vi "acelerometro.vi"(0 "Handle table":string[][](array[string]), 5 "COM Bluegiga in":refnum<visa-resource-name>, 7 "Service UUID":string, 9 "error in (no error)":errorcluster, 11 "Characteristic UUID":string, 12 "Connection Status":T1={"MAC Address"="", "cnx handle"=0, "cnx flags"=0, "Address Type"=125, "Connection Interval (ms)"=125, "Timeout(ms)"=125, "Latency"=0, "bonding handle"=0} {"Address Type" items=["Public", "Random"]}) -> (1 "error out":errorcluster, 3 "COM Bluegiga out":refnum<visa-resource-name>, 6 "z (acel)":dbl, 10 "y (acel)":dbl, 15 "x (acel)":dbl)   [LabVIEW 2020]
uses:
  <vilib>/BLE/type_def/connection_status_bundle.ctl
  <vilib>/BLE/type_def/address_type.ctl
panel:
  out "characteristic value":u8[](array[numeric])
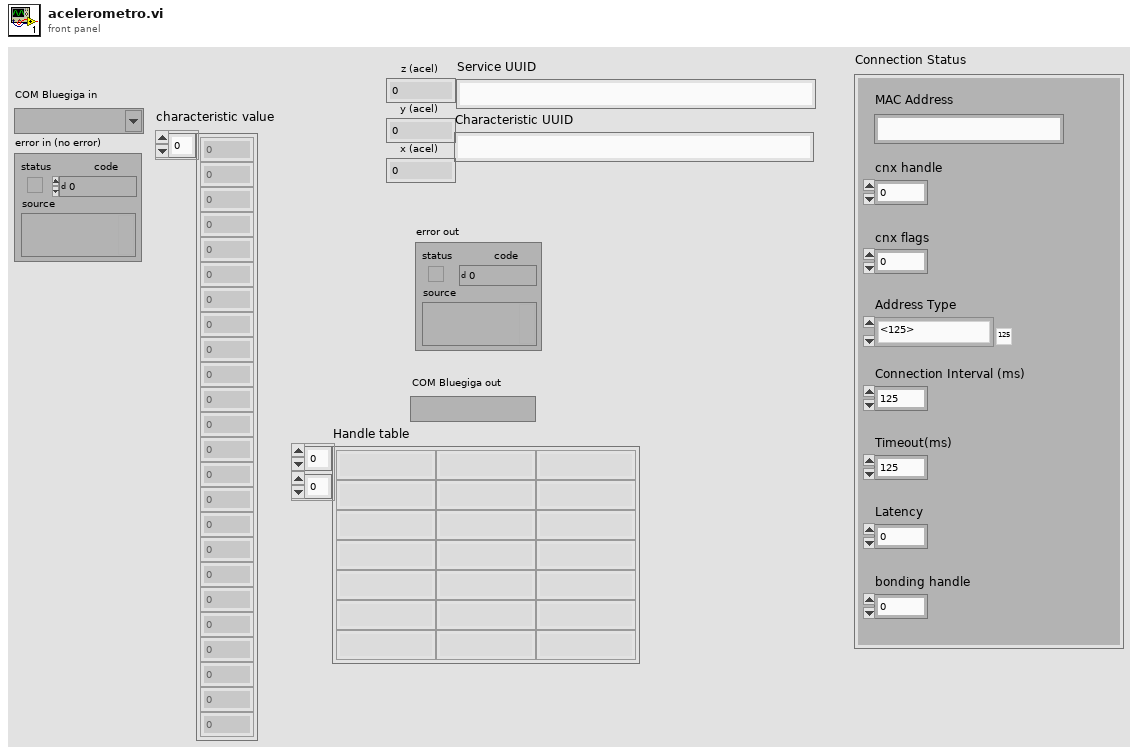
[diagram p1: front panel]
types:
  T1 = typedef "connection_status_bundle.ctl" = cluster{"MAC Address":string, "cnx handle":u8, "cnx flags":u8, "Address Type":T2, "Connection Interval (ms)":u16, "Timeout(ms)":u16, "Latency":u16, "bonding handle":u8}
  T2 = typedef "address_type.ctl" = u8
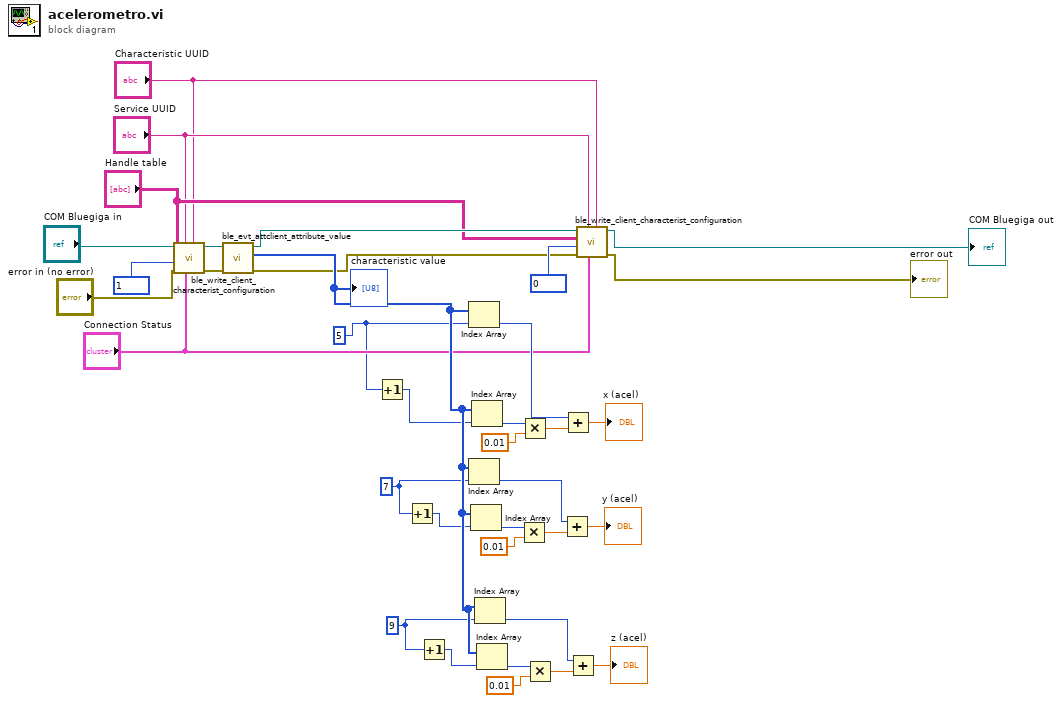
[diagram p0: block diagram]
diagram:
  w1 = 9 ("y")
  w2 = 7 ("y")
  w5 = 5 ("y")
  n1 = call <vilib>:"ble_write_client_characterist_configuration.vi"("Characteristic UUID"="Characteristic UUID", "Connection Status"="Connection Status", "Service UUID"="Service UUID", "error in (no error)"="error in (no error)", "Value(16bit)"=u16 1, "Handle table"="Handle table", "COM Bluegiga in"="COM Bluegiga in") -> ("error out"=w18:errorcluster, "COM Bluegiga out"=w17:refnum<visa-resource-name>)  [unwired: 3 in]
  n2 = call <vilib>:"ble_evt_attclient_attribute_value.vi"("error in (no error)"=w18, "COM Bluegiga in"=w17) -> ("error out"=w13:errorcluster, "characteristic value"=w21:u8[], "COM Bluegiga out"=w14:refnum<visa-resource-name>)  [unwired: 6 in, 1 out]
  "characteristic value" <- w21
  n3 = Increment(x=w5) -> (x+1=w6:i32)
  n4 = Increment(x=w2) -> (x+1=w3:i32)
  n5 = Increment(x=w1) -> (x+1=w4:i32)
  n6 = Index Array(array=w21, index=w5) -> (element=w33:u8)
  n7 = Index Array(array=w21, index=w2) -> (element=w27:u8)
  n8 = Index Array(array=w21, index=w3) -> (element=w28:u8)
  n9 = Index Array(array=w21, index=w6) -> (element=w36:u8)
  n10 = Index Array(array=w21, index=w1) -> (element=w22:u8)
  n11 = Index Array(array=w21, index=w4) -> (element=w23:u8)
  n12 = Multiply(x=w28, y=0.01) -> (x*y=w30:dbl)
  n13 = Multiply(x=w36, y=0.01) -> (x*y=w34:dbl)
  n14 = Multiply(x=w23, y=0.01) -> (x*y=w25:dbl)
  n15 = Add(x=w27, y=w30) -> (x+y=→"y (acel)":dbl)
  n16 = Add(x=w33, y=w34) -> (x+y=→"x (acel)":dbl)
  n17 = Add(x=w22, y=w25) -> (x+y=→"z (acel)":dbl)
  n18 = call <vilib>:"ble_write_client_characterist_configuration.vi"("Characteristic UUID"="Characteristic UUID", "Connection Status"="Connection Status", "Service UUID"="Service UUID", "error in (no error)"=w13, "Value(16bit)"=u16 0, "Handle table"="Handle table", "COM Bluegiga in"=w14) -> ("error out"=→"error out":errorcluster, "COM Bluegiga out"=→"COM Bluegiga out":refnum<visa-resource-name>)  [unwired: 3 in]
